vi "VoltageUpdate.Write Configuration.vi"(8 "error in (no error)":errorcluster, 10 "Configuration":T1, 11 "VoltageUpdate":refnum<class "VoltageUpdate.lvclass">) -> (0 "error out":errorcluster, 3 "VoltageUpdate out":refnum<class "VoltageUpdate.lvclass">)   [LabVIEW 2016, in "VoltageUpdate.lvclass"]
uses:
  VoltageUpdate.lvclass
  Typedefs/VoltageUpdate.Configuration--Cluster.ctl
  VoltageUpdate.lvclass/VoltageUpdate.ctl
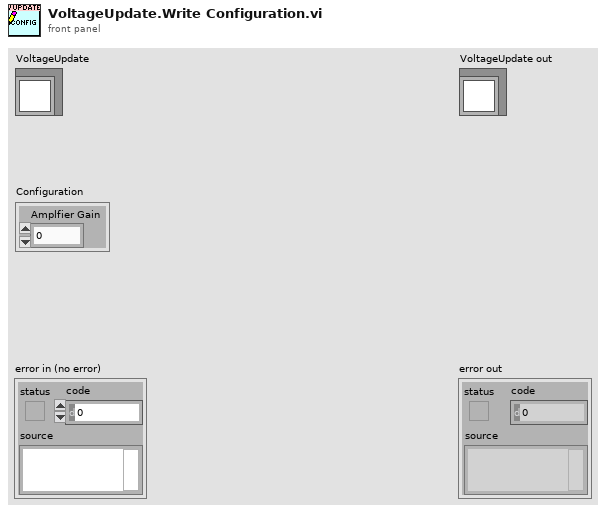
[diagram p1: front panel]
types:
  T1 = typedef "VoltageUpdate.lvclass/VoltageUpdate.Configuration--Cluster.ctl" = cluster{"Amplfier Gain":dbl}
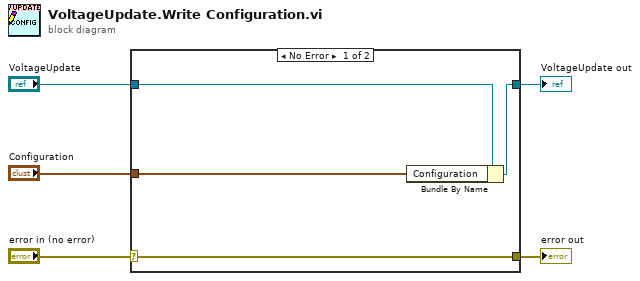
[diagram p0: block diagram]
diagram:
  n1 = case shown="No Error" "error in (no error)" {
    selector: "error in (no error)" -> [w9 w10]
    tunnel: [w9 w10] -> w4
    tunnel: [w7 w11] -> w2
    tunnel: "VoltageUpdate" -> [w8 w11]
    tunnel: "Configuration" -> [w6 _]
    frame No Error {
      n2 = Bundle By Name(cluster=w8, "Configuration"=w6) -> (w7:refnum<class "VoltageUpdate.lvclass">)
    }
    frame Error {
    }
  }
  "error out" <- w4
  "VoltageUpdate out" <- w2
